vi "Write Connection Error.vi"(10 "Connection Error":errorcluster, 11 "AF Queue Stream in":refnum<class "AF Queue Stream.lvclass">) -> (3 "AF Queue Stream out":refnum<class "AF Queue Stream.lvclass">)   [LabVIEW 2020, in "AF Queue Stream.lvclass"]
uses:
  AF Queue Stream.lvclass
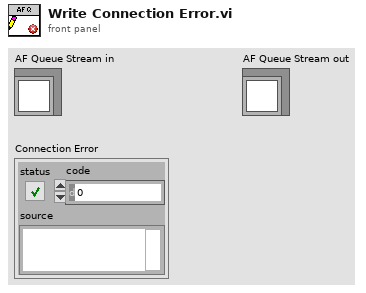
[diagram p1: front panel]
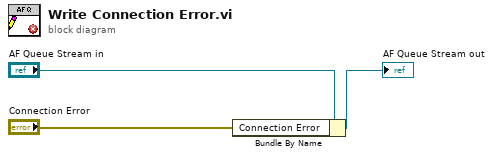
[diagram p0: block diagram]
diagram:
  n1 = Bundle By Name(cluster="AF Queue Stream in", "Connection Error"="Connection Error") -> (→"AF Queue Stream out":refnum<class "AF Queue Stream.lvclass">)
